vi "TL behavior get unstuck_D.vi"(2 "Behavior\nVelocity":dbl, 3 "Activate?":bool=TRUE, 4 "Numeric 2":dbl, 5 "Sensor":T1=[{"Name"="bow", "Angle"=20.0, "Distance"=0.0}, {"Name"="pbow", "Angle"=60.0, "Distance"=0.0}, {"Name"="port", "Angle"=0.0, "Distance"=0.0}, {"Name"="sbow", "Angle"=60.0, "Distance"=0.0}, {"Name"="starboard", "Angle"=0.0, "Distance"=0.0}]) -> (0 "Unstuck Array":dbl[](array[numeric]), 1 "Numeric":dbl)   [LabVIEW 2014]
uses:
  sensorsSTD.ctl
panel:
  out "Waveform Graph":cluster{dbl, dbl, dbl[]}(graph)
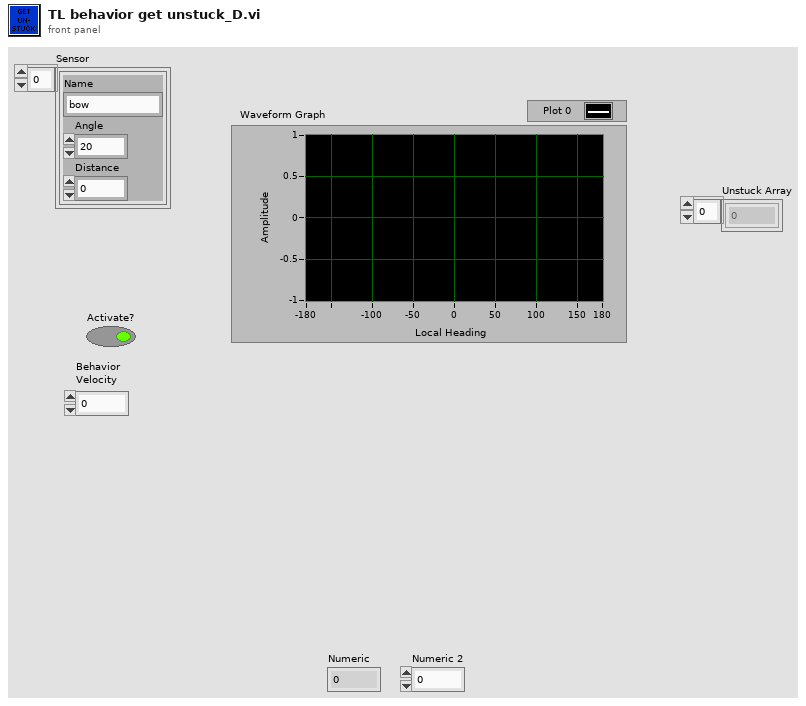
[diagram p1: front panel]
types:
  T1 = typedef "sensorsSTD.ctl" = cluster{"Name":string, "Angle":dbl, "Distance":dbl}[]
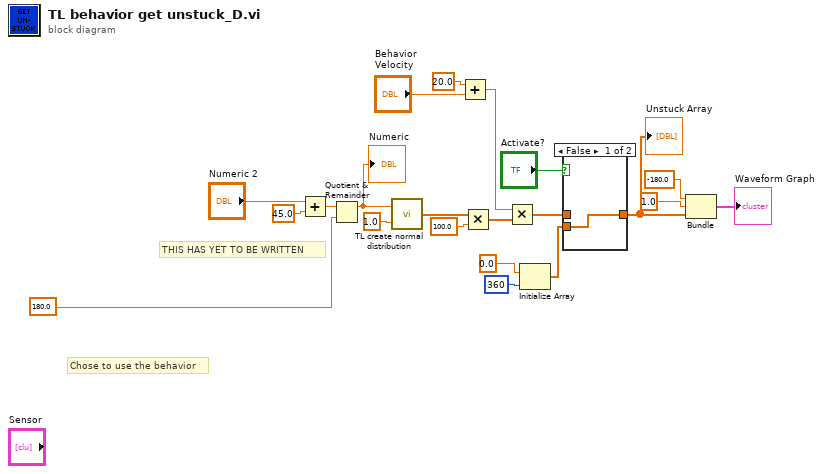
[diagram p0: block diagram]
diagram:
  # "THIS HAS YET TO BE WRITTEN"
  # "Chose to use the behavior"
  n1 = Add(x="Numeric 2", y=45.0 ("std (Normal)")) -> (x+y=w9:dbl)
  n2 = Quotient & Remainder(x=w9, y=180.0 ("std (Normal)")) -> (x-y*floor(x/y)=w7:dbl)  [unwired: 1 out]
  "Numeric" <- w7
  n3 = call "TL create normal distribution.vi"("std (Normal)"=1.0, "mean"=w7) -> ("ACT array"=w3:dbl[])
  n4 = Add(x=20.0 ("std (Normal)"), y="Behavior\nVelocity") -> (x+y=w6:dbl)
  n5 = Multiply(x=w3, y=100.0 ("std (Normal)")) -> (x*y=w2:dbl[])
  n6 = Multiply(x=w6, y=w2) -> (x*y=w12:dbl[])
  n7 = Initialize Array(0.0 ("element"), 360 ("dimension size")) -> (w15:dbl[])
  n8 = case shown="False" "Activate?" {
    tunnel: w15 -> [w22 _]
    tunnel: w12 -> [_ w23]
    tunnel: [w22 w23] -> w14
    frame False {
    }
    frame True {
    }
  }
  "Unstuck Array" <- w14
  n9 = Bundle(-180.0, 1.0, w14) -> (→"Waveform Graph":cluster{dbl, dbl, dbl[]})  [unwired: 1 in]
